vi "Main.vi"() -> ()   [LabVIEW 2013]
uses:
  <vilib>/vision/Image Controls.llb/IMAQ Image.ctl
  Controls/Tip.ctl
  Controls/Track.ctl
  <vilib>/vision/NI_Vision_Development_Module.lvlib
panel:
  in  "Tip Matching Options":T1
  in  "Track Classifier":path
  in  "Tracks":T2[](array[typedef]) {"ROI Descriptor"."Contours"."Type" items=["No Selection", "Point", "Line", "Rectangle", "Oval", "Polygon", "Freehand Region", "Annulus", "Unused2", "Unused3", "Broken Line", "Freehand Line", "Rotated Rectangle"]; "Tip 2"."ROI Descriptor"."Contours"."Type" items=["No Selection", "Point", "Line", "Rectangle", "Oval", "Polygon", "Freehand Region", "Annulus", "Unused2", "Unused3", "Broken Line", "Freehand Line", "Rotated Rectangle"]; "Tip 2"."Point"."Y" format="%.2f"; "Tip 2"."Point"."X" format="%.2f"; "Tip 1"."ROI Descriptor"."Contours"."Type" items=["No Selection", "Point", "Line", "Rectangle", "Oval", "Polygon", "Freehand Region", "Annulus", "Unused2", "Unused3", "Broken Line", "Freehand Line", "Rotated Rectangle"]; "Tip 1"."Point"."Y" format="%.2f"; "Tip 1"."Point"."X" format="%.2f"}
  in  "Flattened Stack":T6
  in  "Tip Classifier":path
  in  "Tips":T3[](array[typedef]) {"ROI Descriptor"."Contours"."Type" items=["No Selection", "Point", "Line", "Rectangle", "Oval", "Polygon", "Freehand Region", "Annulus", "Unused2", "Unused3", "Broken Line", "Freehand Line", "Rotated Rectangle"]; "Point"."Y" format="%.2f"; "Point"."X" format="%.2f"}
  in  "Tab Control":enum32{"Tip Extraction", "Track Extraction"}(tab)
  in  "Classify Tips":bool
  in  "Find Potential Tips":bool
  out "Progress":u8(slide) scale=0.0..100.0
  in  "Save Samples":bool
  in  "Reset":bool
  in  "Process AVI":bool
  in  "Process Directory":bool
  out "Currently Processing:":string
  in  "Stop":bool
  in  "Skip":bool
  out "Files to Process":i32
  in  "Tip Destination":path=path "C:/Users/Andrew/Documents/Apatite to Zircon Code/Track Finding/Tip Images/Tips/unprocessed"
  in  "Non-tip Destination":path=path "C:/Users/Andrew/Documents/Apatite to Zircon Code/Track Finding/Tip Images/Non-Tips/unprocessed"
  out "Tip Image":T6(plugin-control)
  in  "Save Track Samples":bool
  in  "Skip Track":bool
  in  "Track -":bool
  in  "Track +":bool
  in  "Classify Tracks":bool
  in  "Match Tips":bool
  in  "Track Destination":path=path "C:/Users/Andrew/Documents/Apatite to Zircon Code/Track Finding/Track Images/Tracks/unprocessed"
  in  "Non-track Destination":path=path "C:/Users/Andrew/Documents/Apatite to Zircon Code/Track Finding/Track Images/Non-tracks/unprocessed"
  out "Selected Track":T6(plugin-control)
  in  "Candidate Tracks":i32(listbox)
  out "File Index":i32
  in  "Image Array":T6[](array[typedef])
  in  "Filenames":path[](array[path])
  in  "Frame":i32(slide)
  in  "Current Image":T6(plugin-control)
  out "error out":errorcluster
  in  "error in (no error)":errorcluster
  # "AVI Processing"
  # "Extracted Samples"
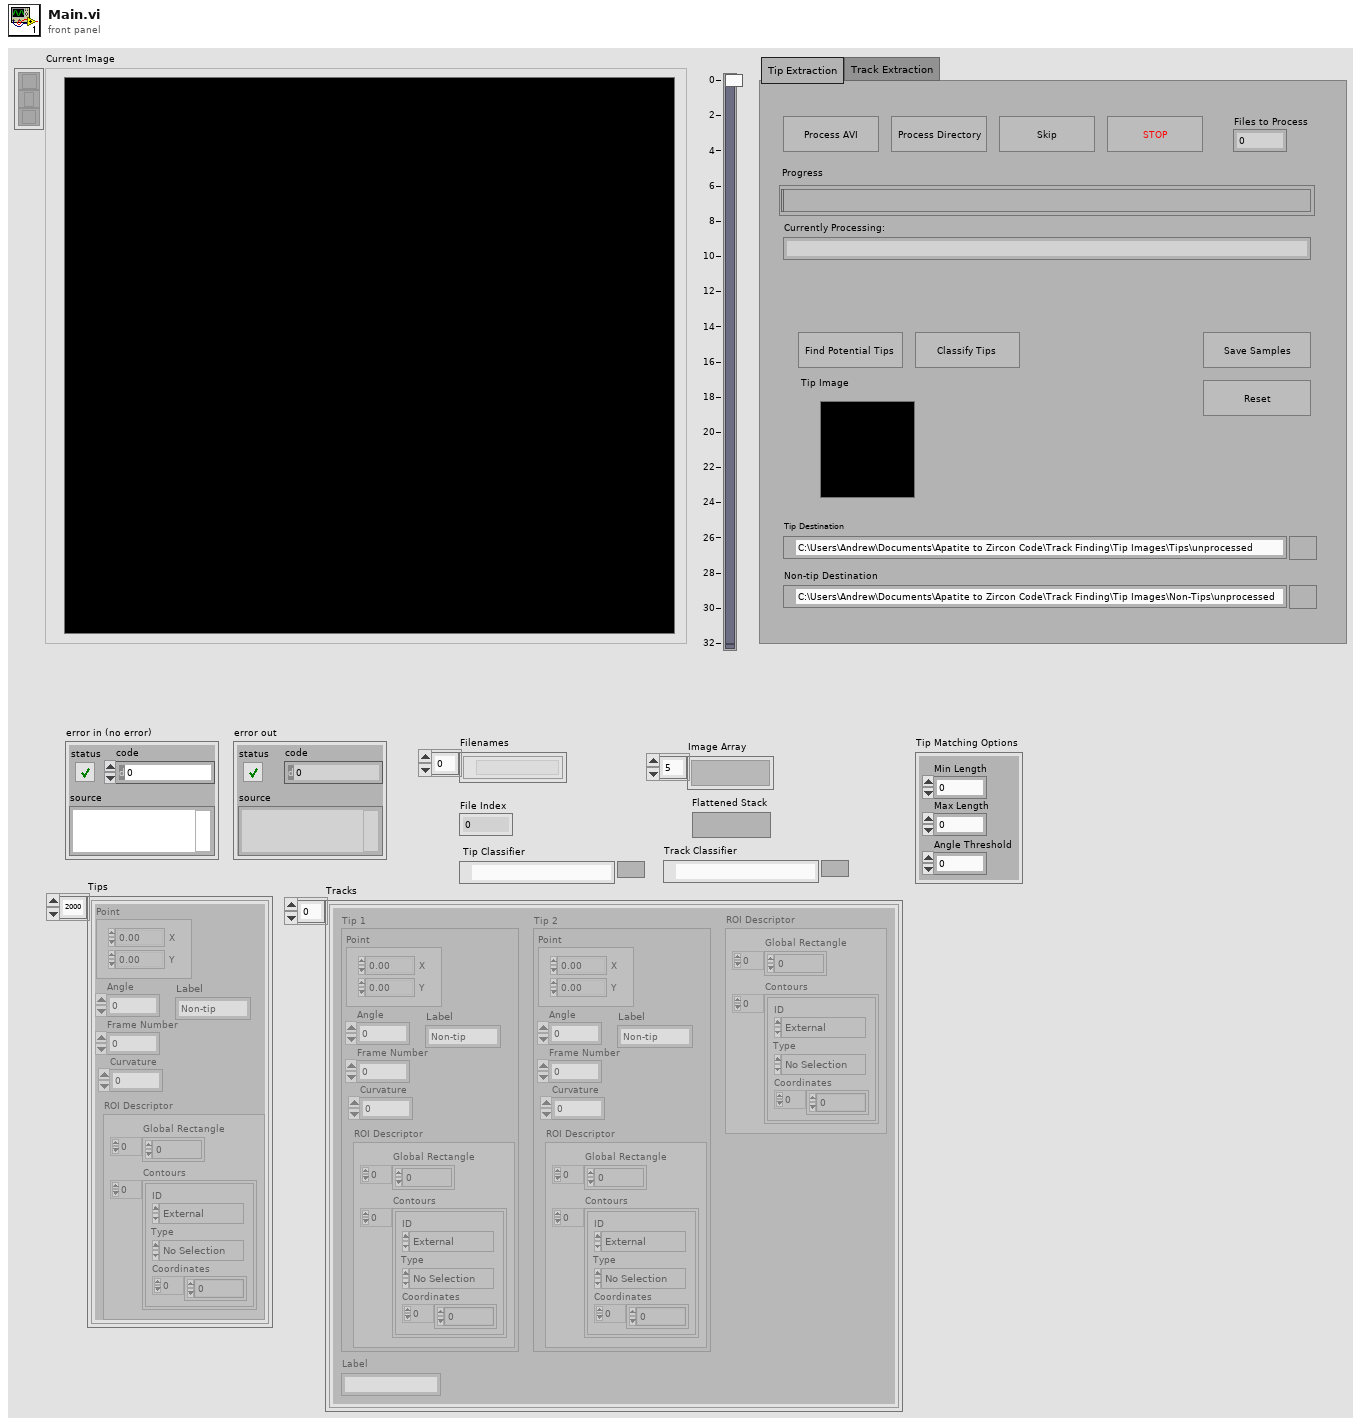
[diagram p1: front panel]
types:
  T1 = cluster{"Min Length":dbl, "Max Length":dbl, "Angle Threshold":dbl}
  T2 = typedef "Track.ctl" = cluster{"Tip 1":T3, "Tip 2":T3, "Label":string, "ROI Descriptor":T5}
  T3 = typedef "Tip.ctl" = cluster{"Point":T4, "Angle":dbl, "Frame Number":i32, "ROI Descriptor":T5, "Curvature":dbl, "Label":string}
  T4 = typedef "IMAQ Point" = cluster{"X":sgl, "Y":sgl}
  T5 = typedef "ROI Descriptor" = cluster{"Global Rectangle":i32[], "Contours":cluster{"ID":enum32{"External", "Internal"}, "Type":u32, "Coordinates":i32[]}[]}
  T6 = typedef "IMAQ Image.ctl" = refnum<image>
  T7 = enum8{"Enabled", "Disabled", "Disabled and Grayed Out"}
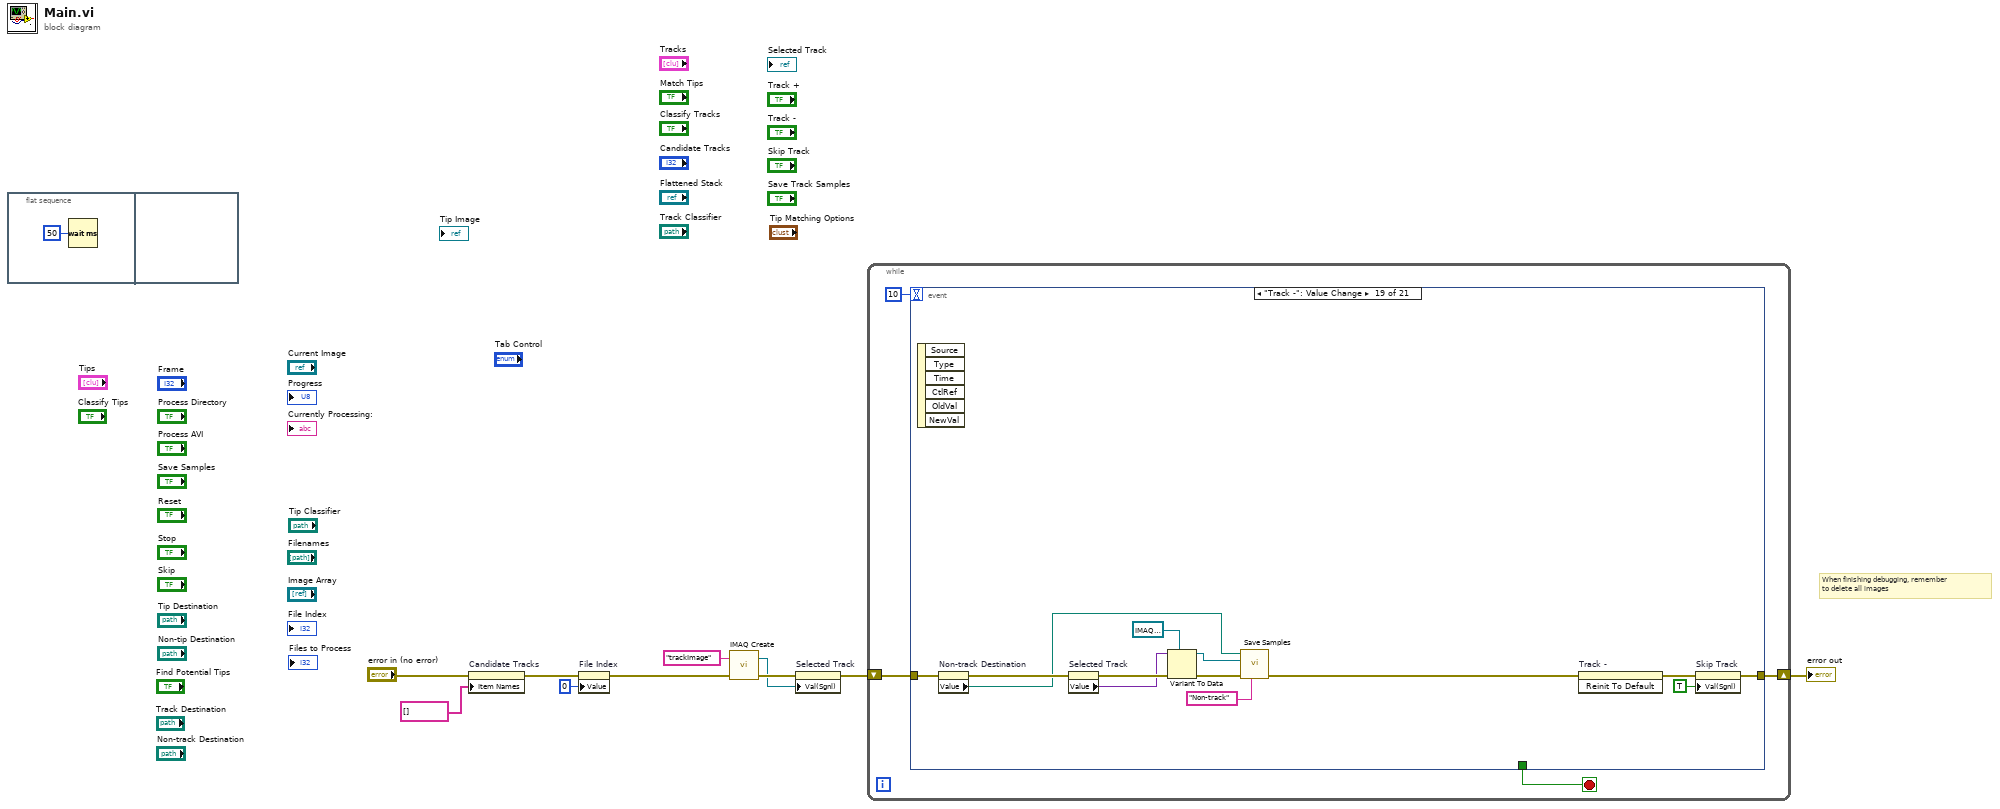
[diagram p0: block diagram]
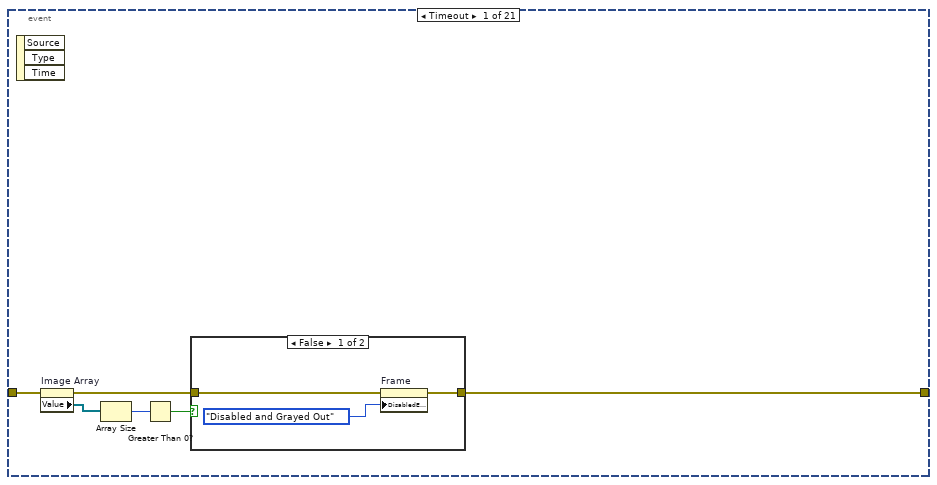
[diagram p2: hidden frame]
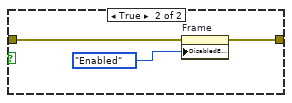
[diagram p3: hidden frame]
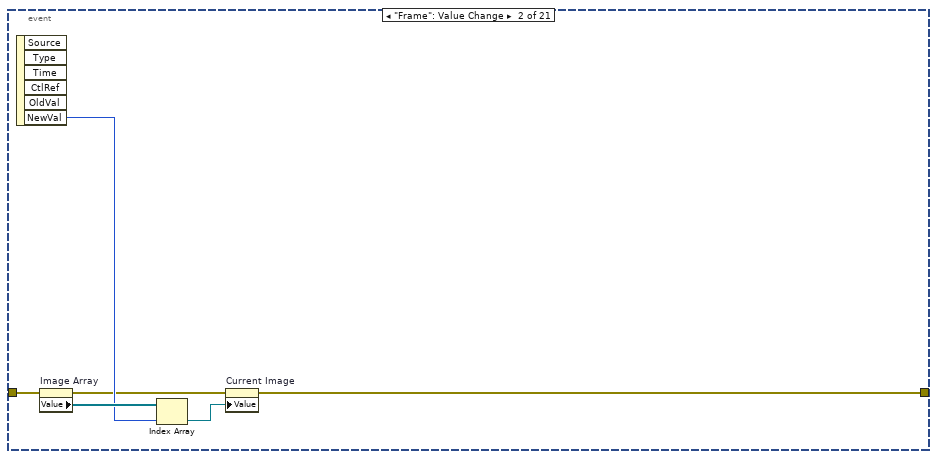
[diagram p4: hidden frame]
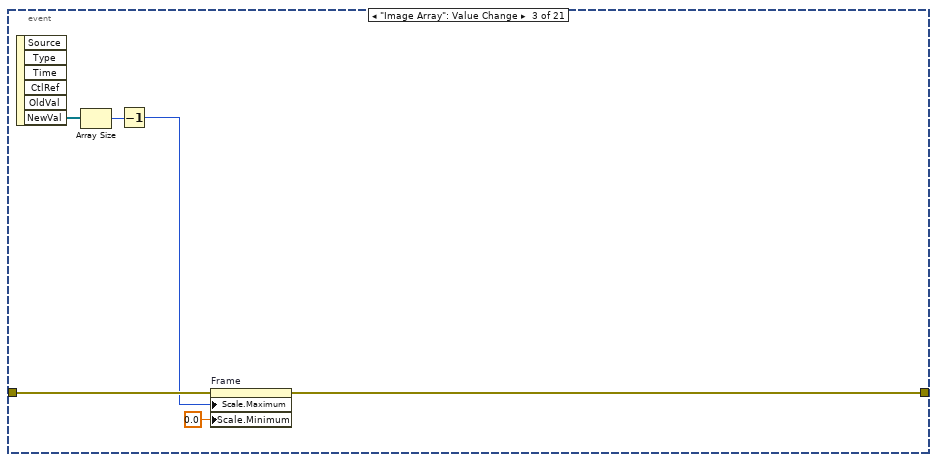
[diagram p5: hidden frame]
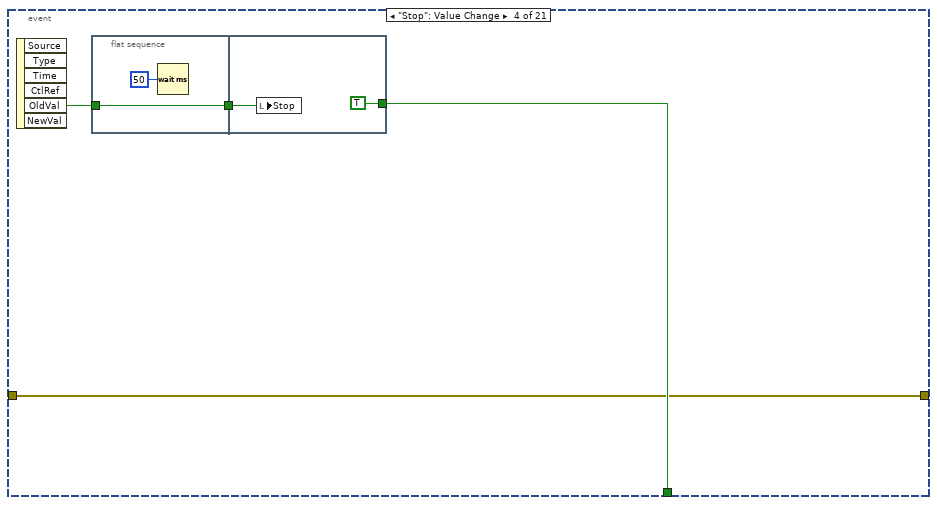
[diagram p6: hidden frame]
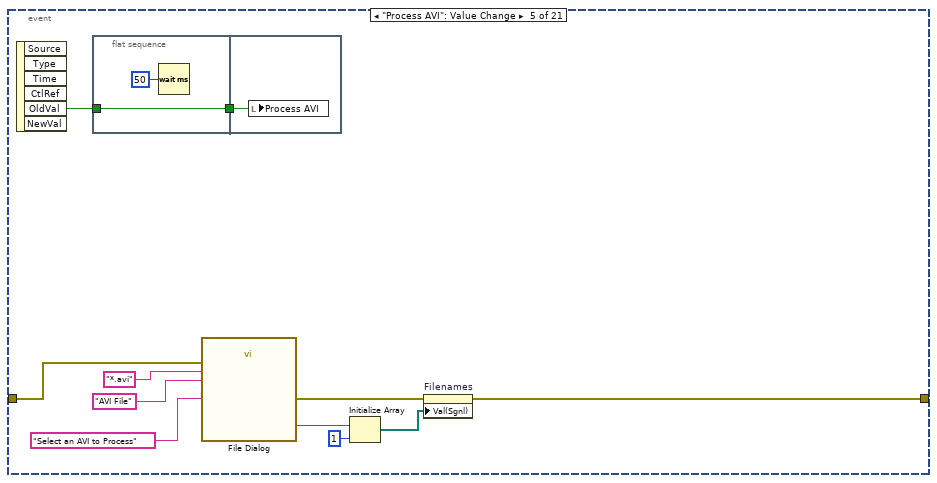
[diagram p7: hidden frame]
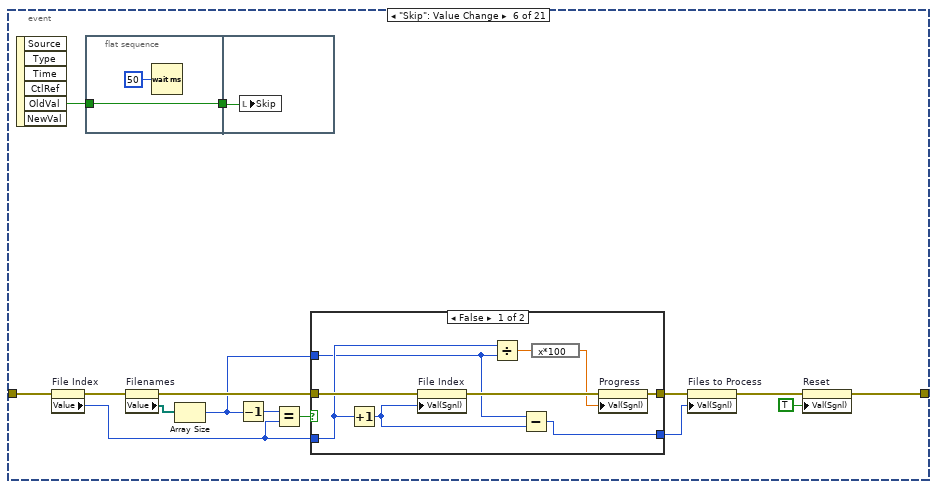
[diagram p8: hidden frame]
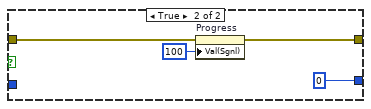
[diagram p9: hidden frame]
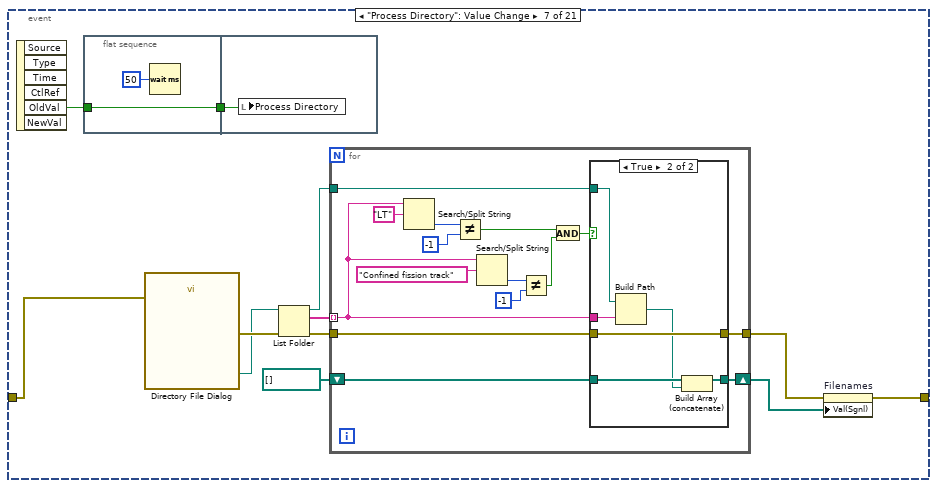
[diagram p10: hidden frame]
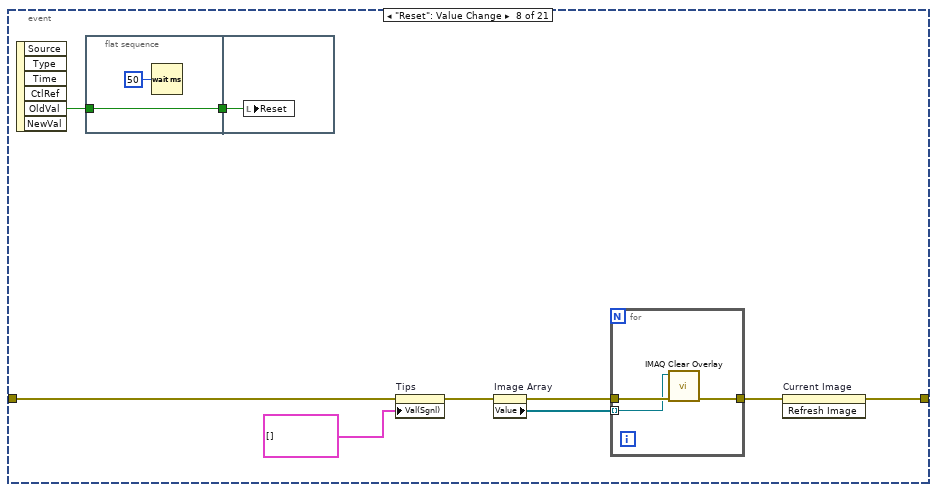
[diagram p12: hidden frame]
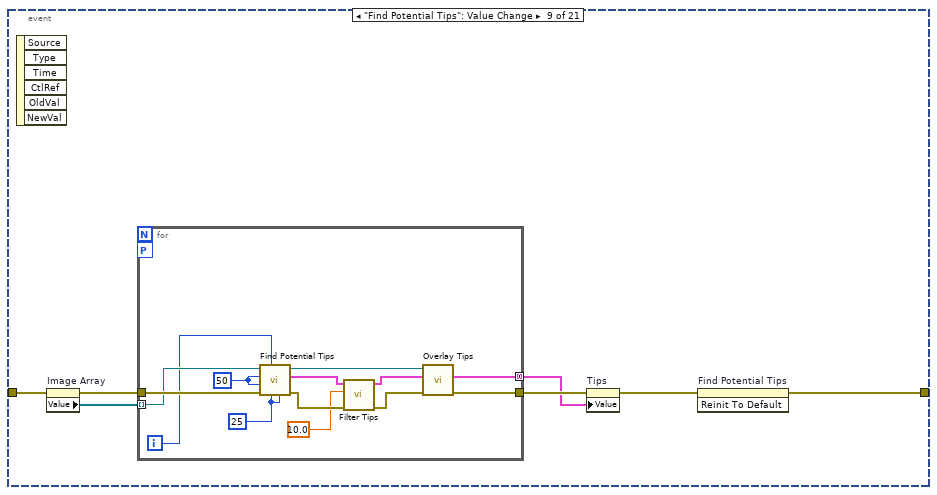
[diagram p13: hidden frame]
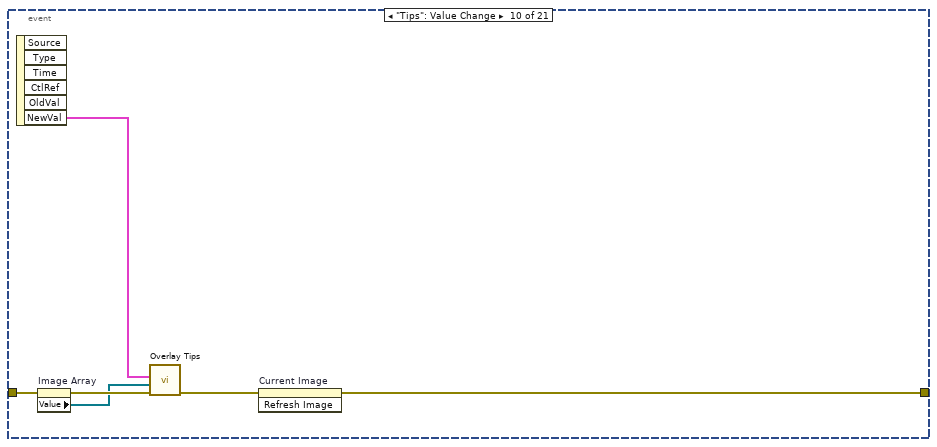
[diagram p14: hidden frame]
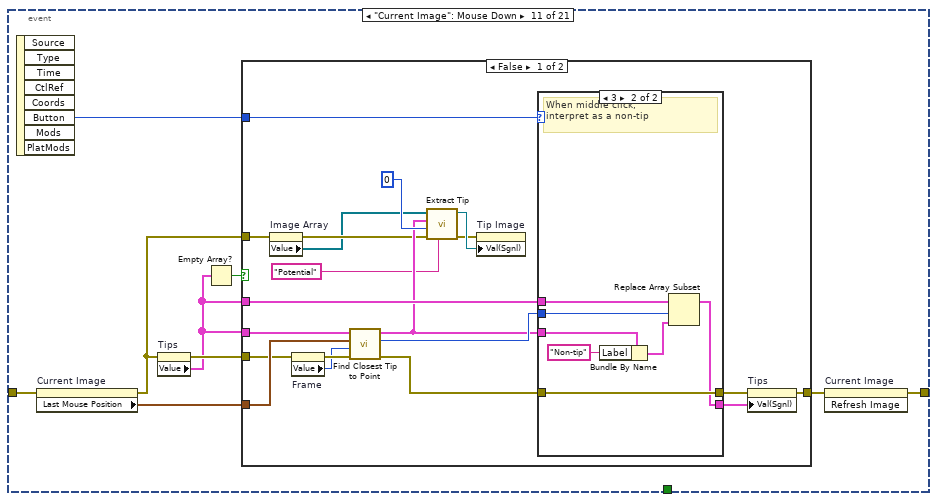
[diagram p15: hidden frame]
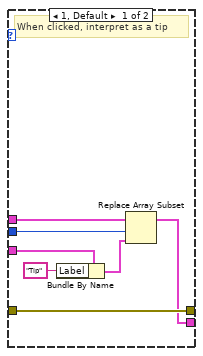
[diagram p16: hidden frame]
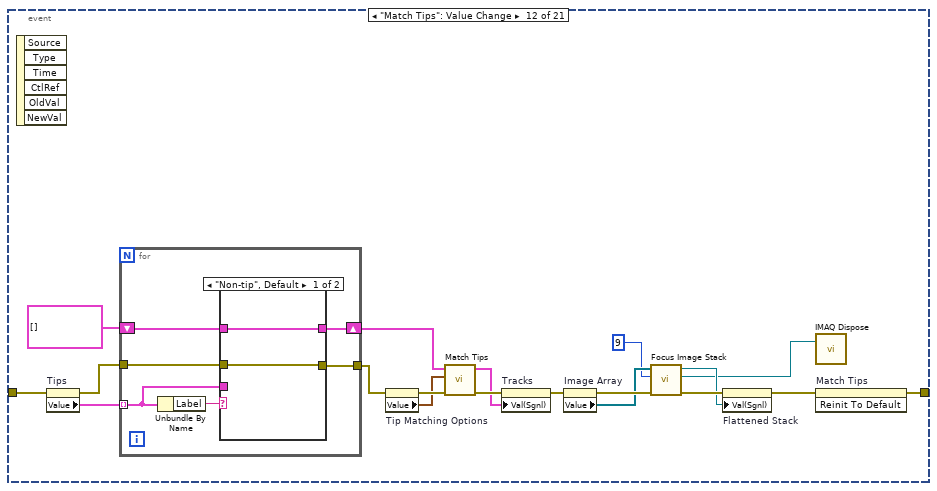
[diagram p18: hidden frame]
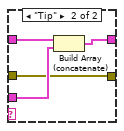
[diagram p19: hidden frame]
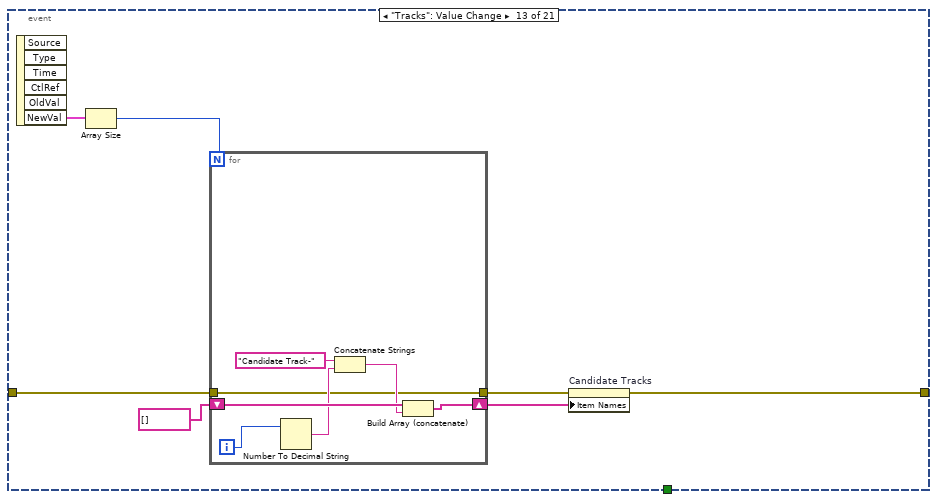
[diagram p20: hidden frame]
diagram:
  # "When finishing debugging, remember \nto delete all images"
  n1 = flat-sequence {
    frame #0 {
      n2 = Wait (ms)(milliseconds to wait=u32 50) -> ()  [unwired: 1 out]
    }
    frame #1 {
    }
  }
  n3 = property on="Candidate Tracks" class="LstBox (strict)"(error in="error in (no error)", "Item Names"=string[] []) -> (error out=w7:errorcluster)  [unwired: 1 in, 1 out]
  n4 = property on="File Index" class="DigNum (strict)"(error in=w7, "Value"=0 ("File Index")) -> (error out=w4:errorcluster)  [unwired: 1 in, 1 out]
  n5 = call "IMAQ Create"("Image Name"="trackImage", "error in (no error)"=w4) -> ("New Image"=w2:T6, "error out"=w3:errorcluster)  [unwired: 3 in]
  n6 = property on="Selected Track" class="ImageControl"(error in=w3, "Val(Sgnl)"=w2) -> (error out=w1:errorcluster)  [unwired: 1 in, 1 out]
  n7 = while {
    shift-right: [w13] -> w10
    shift-left: w1 -> [w14]
    stop <- w15 stop-if-true
    n8 = event shown="[18] \"Track -\": Value Change" {
      selector: _ -> [_ _ _ _ _ _ _ _ _ _ _ _ _ _ _ _ _ _ _ _ _]
      dyn-events: _ -> [_ _ _ _ _ _ _ _ _ _ _ _ _ _ _ _ _ _ _ _ _]
      timeout: 10 -> [_ _ _ _ _ _ _ _ _ _ _ _ _ _ _ _ _ _ _ _ _]
      tunnel: [_ _ _ w41 _ _ _ _ _ _ _ _ _ _ _ _ _ _ _ _ _] -> w15
      tunnel: w14 -> [w21 w33 w39 w40 w56 w74 w102 w132 w152 w171 w180 w231 w248 w279 w289 w304 w317 w364 w377 w386 w394]
      tunnel: [w16 w28 w35 w40 w49 w63 w97 w134 w146 w166 w177 w234 w249 w266 w280 w305 w319 w367 w380 w381 w387] -> w13
      event Timeout {
        n9 = event-data() -> ()  [unwired: 1 in, 3 out]
        n10 = property on="Image Array" class="Arr (strict)"(error in=w21) -> (error out=w17:errorcluster, "Value"=w20:T6[])  [unwired: 1 in, 1 out]
        n11 = Array Size(array=w20) -> (size(s)=w19:i32)
        n12 = Greater Than 0?(x=w19) -> (x > 0?=w18:bool)
        n13 = case shown="False" w18 {
          tunnel: w17 -> [w24 w26]
          tunnel: [w23 w25] -> w16
          frame False {
            n14 = property on="Frame" class="Slide (strict)"(error in=w24, "DisabledEnum"=T7."Disabled and Grayed Out" ("Disabled")) -> (error out=w23:errorcluster)  [unwired: 1 in, 1 out]
          }
          frame True {
            n15 = property on="Frame" class="Slide (strict)"(error in=w26, "DisabledEnum"=T7."Enabled" ("Disabled")) -> (error out=w25:errorcluster)  [unwired: 1 in, 1 out]
          }
        }
      }
      event "Frame": Value Change {
        n16 = event-data() -> ("NewVal"=w31:i32)  [unwired: 1 in, 5 out]
        n17 = property on="Image Array" class="Arr (strict)"(error in=w33) -> (error out=w30:errorcluster, "Value"=w32:T6[])  [unwired: 1 in, 1 out]
        n18 = Index Array(array=w32, index=w31) -> (element=w29:T6)
        n19 = property on="Current Image" class="ImageControl"(error in=w30, "Value"=w29) -> (error out=w28:errorcluster)  [unwired: 1 in, 1 out]
      }
      event "Image Array": Value Change {
        n20 = event-data() -> ("NewVal"=w38:T6[])  [unwired: 1 in, 5 out]
        n21 = Array Size(array=w38) -> (size(s)=w37:i32)
        n22 = Decrement(x=w37) -> (x-1=w36:i32)
        n23 = property on="Frame" class="Slide (strict)"(error in=w39, "Scale.Maximum"=w36, "Scale.Minimum"=0.0 ("Scale.Range:Minimum")) -> (error out=w35:errorcluster)  [unwired: 1 in, 1 out]
      }
      event "Stop": Value Change {
        n24 = event-data() -> ("OldVal"=w43:bool)  [unwired: 1 in, 5 out]
        n25 = flat-sequence {
          tunnel: w43 -> [w44]
          tunnel: [w44] -> w42
          tunnel: w42 -> [w47]
          tunnel: [TRUE] -> w41
          frame #0 {
            n26 = Wait (ms)(milliseconds to wait=u32 50) -> ()  [unwired: 1 out]
          }
          frame #1 {
            n27 = local write "Stop"(w47) -> ()
          }
        }
      }
      event "Process AVI": Value Change {
        n28 = event-data() -> ("OldVal"=w58:bool)  [unwired: 1 in, 5 out]
        n29 = flat-sequence {
          tunnel: w58 -> [w59]
          tunnel: [w59] -> w57
          tunnel: w57 -> [w61]
          frame #0 {
            n30 = Wait (ms)(milliseconds to wait=u32 50) -> ()  [unwired: 1 out]
          }
          frame #1 {
            n31 = local write "Process AVI"(w61) -> ()
          }
        }
        n32 = call "File Dialog"("prompt"="Select an AVI to Process", "error in"=w56, "pattern (all files)"="*.avi", "pattern label"="AVI File") -> ("selected path"=w53:path, "error out"=w50:errorcluster)  [unwired: 8 in, 2 out]
        n33 = Initialize Array(w53, 1 ("dimension size")) -> (w51:path[])
        n34 = property on="Filenames" class="Arr (strict)"(error in=w50, "Val(Sgnl)"=w51) -> (error out=w49:errorcluster)  [unwired: 1 in, 1 out]
      }
      event "Skip": Value Change {
        n35 = event-data() -> ("OldVal"=w75:bool)  [unwired: 1 in, 5 out]
        n36 = property on="File Index" class="DigNum (strict)"(error in=w74) -> (error out=w73:errorcluster, "Value"=w69:i32)  [unwired: 1 in, 1 out]
        n37 = flat-sequence {
          tunnel: [w90] -> w76
          tunnel: w75 -> [w90]
          tunnel: w76 -> [w92]
          frame #0 {
            n38 = Wait (ms)(milliseconds to wait=u32 50) -> ()  [unwired: 1 out]
          }
          frame #1 {
            n39 = local write "Skip"(w92) -> ()
          }
        }
        n40 = property on="Filenames" class="Arr (strict)"(error in=w73) -> (error out=w71:errorcluster, "Value"=w72:path[])  [unwired: 1 in, 1 out]
        n41 = Array Size(array=w72) -> (size(s)=w67:i32)
        n42 = Decrement(x=w67) -> (x-1=w68:i32)
        n43 = Equal?(x=w68, y=w69) -> (x = y?=w70:bool)
        n44 = case shown="False" w70 {
          tunnel: w71 -> [w85 w89]
          tunnel: w69 -> [w79 _]
          tunnel: [w83 w88] -> w66
          tunnel: w67 -> [w77 _]
          tunnel: [w78 0] -> w65
          frame False {
            n45 = Increment(x=w79) -> (x+1=w80:i32)
            n46 = property on="File Index" class="DigNum (strict)"(error in=w85, "Val(Sgnl)"=w80) -> (error out=w84:errorcluster)  [unwired: 1 in, 1 out]
            n47 = Divide(x=w79, y=w77) -> (x/y=w82:dbl)
            n48 = Subtract(x=w77, y=w80) -> (x-y=w78:i32)
            n49 = expression code="x*100"(w82) -> (w81:dbl)
            n50 = property on="Progress" class="Slide (strict)"(error in=w84, "Val(Sgnl)"=w81) -> (error out=w83:errorcluster)  [unwired: 1 in, 1 out]
          }
          frame True {
            n51 = property on="Progress" class="Slide (strict)"(error in=w89, "Val(Sgnl)"=u8 100 ("Value (Signaling)")) -> (error out=w88:errorcluster)  [unwired: 1 in, 1 out]
          }
        }
        n52 = property on="Files to Process" class="DigNum (strict)"(error in=w66, "Val(Sgnl)"=w65) -> (error out=w64:errorcluster)  [unwired: 1 in, 1 out]
        n53 = property on="Reset" class="Bool (strict)"(error in=w64, "Val(Sgnl)"=TRUE ("Value (Signaling)")) -> (error out=w63:errorcluster)  [unwired: 1 in, 1 out]
      }
      event "Process Directory": Value Change {
        n54 = event-data() -> ("OldVal"=w104:bool)  [unwired: 1 in, 5 out]
        n55 = flat-sequence {
          tunnel: w104 -> [w128]
          tunnel: [w128] -> w103
          tunnel: w103 -> [w130]
          frame #0 {
            n56 = Wait (ms)(milliseconds to wait=u32 50) -> ()  [unwired: 1 out]
          }
          frame #1 {
            n57 = local write "Process Directory"(w130) -> ()
          }
        }
        n58 = call "Directory File Dialog"("error in"=w102) -> ("selected path"=w98:path, "error out"=w99:errorcluster)  [unwired: 11 in, 2 out]
        n59 = List Folder(path=w98, error in=w99) -> (path out=w96:path, filenames=w101:string[], error out=w100:errorcluster)  [unwired: 2 in, 1 out]
        n60 = for {
          tunnel: w101 -> [w108] mode=indexing
          tunnel: w100 -> [w114]
          shift-right: [w115] -> w94
          shift-left: path[] [] -> [w116]
          tunnel: [w113] -> w93
          tunnel: w96 -> [w112]
          n61 = Search/Split String(string=w108, search string/char (-)="LT") -> (offset of match=w119:i32)  [unwired: 1 in, 2 out]
          n62 = Not Equal?(x=w119, y=-1) -> (x != y?=w106:bool)
          n63 = Search/Split String(string=w108, search string/char (-)="Confined fission track") -> (offset of match=w109:i32)  [unwired: 1 in, 2 out]
          n64 = Not Equal?(x=w109, y=-1) -> (x != y?=w107:bool)
          n65 = And(x=w106, y=w107) -> (x .and. y?=w105:bool)
          n66 = case shown="True" w105 {
            tunnel: w116 -> [w120 w127]
            tunnel: [w120 w126] -> w115
            tunnel: w108 -> [_ w124]
            tunnel: w114 -> [w121 w125]
            tunnel: [w121 w125] -> w113
            tunnel: w112 -> [_ w123]
            frame False {
            }
            frame True {
              n67 = Build Path(base path=w123, name or relative path=w124) -> (appended path=w122:path)
              n68 = Build Array (concatenate)(w127, w122) -> (w126:path[])
            }
          }
        }
        n69 = property on="Filenames" class="Arr (strict)"(error in=w93, "Val(Sgnl)"=w94) -> (error out=w97:errorcluster)  [unwired: 1 in, 1 out]
      }
      event "Reset": Value Change {
        n70 = event-data() -> ("OldVal"=w139:bool)  [unwired: 1 in, 5 out]
        n71 = flat-sequence {
          tunnel: w139 -> [w143]
          tunnel: [w143] -> w138
          tunnel: w138 -> [w145]
          frame #0 {
            n72 = Wait (ms)(milliseconds to wait=u32 50) -> ()  [unwired: 1 out]
          }
          frame #1 {
            n73 = local write "Reset"(w145) -> ()
          }
        }
        n74 = property on="Tips" class="Arr (strict)"(error in=w132, "Val(Sgnl)"=T3[] [] ("Value (Signaling)")) -> (error out=w133:errorcluster)  [unwired: 1 in, 1 out]
        n75 = property on="Image Array" class="Arr (strict)"(error in=w133) -> (error out=w136:errorcluster, "Value"=w137:T6[])  [unwired: 1 in, 1 out]
        n76 = for {
          tunnel: w137 -> [w141] mode=indexing
          tunnel: w136 -> [w142]
          tunnel: [w140] -> w135
          n77 = call "IMAQ Clear Overlay"("error in (no error)"=w142, "Image"=w141) -> ("error out"=w140:errorcluster)  [unwired: 8 in, 1 out]
        }
        n78 = invoke on="Current Image" class="ImageControl" method="Refresh Image"(error in=w135) -> (error out=w134:errorcluster)  [unwired: 2 in, 2 out]
      }
      event "Find Potential Tips": Value Change {
        n79 = event-data() -> ()  [unwired: 1 in, 6 out]
        n80 = property on="Image Array" class="Arr (strict)"(error in=w152) -> (error out=w151:errorcluster, "Value"=w150:T6[])  [unwired: 1 in, 1 out]
        n81 = for {
          workers-P: _ -> [_]
          tunnel: w151 -> [w165]
          tunnel: w150 -> [w164] mode=indexing
          tunnel: [w154] -> w148 mode=concatenating
          tunnel: [w153] -> w149
          i -> [w163]
          w161 = 50 ("ROI Width")
          w162 = 25 ("dx")
          n82 = call "Find Potential Tips.vi"("dy"=w162, "dx"=w162, "Frame Number"=w163, "error in (no error)"=w165, "ROI Height"=w161, "ROI Width"=w161, "Image"=w164) -> ("error out"=w160:errorcluster, "Potential Tips"=w159:T3[], "Image out"=w155:T6)  [unwired: 2 in]
          n83 = call "Filter Tips.vi"("error in (no error)"=w160, "Duplicate Distance"=10.0, "Tips"=w159) -> ("error out"=w156:errorcluster, "Filtered Tips"=w157:T3[])  [unwired: 7 in]
          n84 = call "Overlay Tips.vi"("error in (no error)"=w156, "Tips"=w157, "Image"=w155) -> ("error out"=w153:errorcluster, "Tips out"=w154:T3[])  [unwired: 6 in, 1 out]
        }
        n85 = property on="Tips" class="Arr (strict)"(error in=w149, "Value"=w148) -> (error out=w147:errorcluster)  [unwired: 1 in, 1 out]
        n86 = invoke on="Find Potential Tips" class="Bool (strict)" method="Reinit To Default"(error in=w147) -> (error out=w146:errorcluster)  [unwired: 2 in, 2 out]
      }
      event "Tips": Value Change {
        n87 = event-data() -> ("NewVal"=w168:T3[])  [unwired: 1 in, 5 out]
        n88 = property on="Image Array" class="Arr (strict)"(error in=w171) -> (error out=w170:errorcluster, "Value"=w169:T6[])  [unwired: 1 in, 1 out]
        n89 = call "Overlay Tips.vi"("error in (no error)"=w170, "Image Array"=w169, "Tips"=w168) -> ("error out"=w167:errorcluster)  [unwired: 6 in, 2 out]
        n90 = invoke on="Current Image" class="ImageControl" method="Refresh Image"(error in=w167) -> (error out=w166:errorcluster)  [unwired: 2 in, 2 out]
      }
      event "Current Image": Mouse Down {
        n91 = event-data() -> ("Button"=w178:u16)  [unwired: 1 in, 7 out]
        n92 = property on="Current Image" class="ImageControl"(error in=w180) -> (error out=w172:errorcluster, "Last Mouse Position"=w179:cluster{"X":i32, "Y":i32})  [unwired: 1 in, 1 out]
        n93 = property on="Tips" class="Arr (strict)"(error in=w172) -> (error out=w175:errorcluster, "Value"=w173:T3[])  [unwired: 1 in, 1 out]
        n94 = Empty Array?(array=w173) -> (empty?=w174:bool)
        n95 = case shown="False" w174 {
          tunnel: w179 -> [w195 _]
          tunnel: w178 -> [w200 _]
          tunnel: [w199 w215] -> w176
          tunnel: w175 -> [w194 w215]
          tunnel: w173 -> [w196 _]
          tunnel: w173 -> [w190 _]
          tunnel: w172 -> [w184 _]
          frame False {
            n96 = property on="Image Array" class="Arr (strict)"(error in=w184) -> (error out=w182:errorcluster, "Value"=w181:T6[])  [unwired: 1 in, 1 out]
            n97 = property on="Frame" class="Slide (strict)"(error in=w194) -> (error out=w193:errorcluster, "Value"=w192:i32)  [unwired: 1 in, 1 out]
            n98 = call "Find Closest Tip to Point.vi"("error in (no error)"=w193, "Frame Number"=w192, "Point"=w195, "Tips"=w196) -> ("error out"=w191:errorcluster, "Tip Index"=w189:i32, "Tip"=w185:T3)  [unwired: 5 in]
            n99 = call "Extract Tip.vi"("Label"="Potential", "error in (no error)"=w182, "Tip Number"=0, "Tip"=w185, "Image Array"=w181) -> ("error out"=w186:errorcluster, "Tip Image"=w187:T6)  [unwired: 5 in]
            n100 = property on="Tip Image" class="ImageControl"(error in=w186, "Val(Sgnl)"=w187) -> ()  [unwired: 1 in, 2 out]
            n101 = case shown="3" w200 {
              tunnel: w191 -> [w207 w214]
              tunnel: [w207 w214] -> w198
              tunnel: [w201 w208] -> w197
              tunnel: w185 -> [w206 w209]
              tunnel: w190 -> [w204 w211]
              tunnel: w189 -> [w203 w210]
              frame 1, Default {
                # "When clicked, interpret as a tip"
                n102 = Bundle By Name(cluster=w206, "Label"="Tip") -> (w202:T3)
                n103 = Replace Array Subset(array=w204, new element=w202, index=w203) -> (w201:T3[])
              }
              frame 3 {
                # "When middle click, \ninterpret as a non-tip"
                n104 = Bundle By Name(cluster=w209, "Label"="Non-tip") -> (w213:T3)
                n105 = Replace Array Subset(array=w211, new element=w213, index=w210) -> (w208:T3[])
              }
            }
            n106 = property on="Tips" class="Arr (strict)"(error in=w198, "Val(Sgnl)"=w197) -> (error out=w199:errorcluster)  [unwired: 1 in, 1 out]
          }
          frame True {
          }
        }
        n107 = invoke on="Current Image" class="ImageControl" method="Refresh Image"(error in=w176) -> (error out=w177:errorcluster)  [unwired: 2 in, 2 out]
      }
      event "Match Tips": Value Change {
        n108 = event-data() -> ()  [unwired: 1 in, 6 out]
        n109 = property on="Tips" class="Arr (strict)"(error in=w231) -> (error out=w228:errorcluster, "Value"=w227:T3[])  [unwired: 1 in, 1 out]
        n110 = for {
          tunnel: w228 -> [w236]
          tunnel: w227 -> [w237] mode=indexing
          shift-right: [w238] -> w224
          shift-left: T3[] [] -> [w239]
          tunnel: [w235] -> w226
          n111 = Unbundle By Name(w237) -> ("Label"=w240:string)
          n112 = case shown="\"Non-tip\", Default" w240 {
            tunnel: w239 -> [w242 w246]
            tunnel: [w242 w245] -> w238
            tunnel: w237 -> [_ w244]
            tunnel: [w241 w243] -> w235
            tunnel: w236 -> [w241 w243]
            frame "Non-tip", Default {
            }
            frame "Tip" {
              n113 = Build Array (concatenate)(w246, w244) -> (w245:T3[])
            }
          }
        }
        n114 = property on="Tip Matching Options" class="Clust (strict)"(error in=w226) -> (error out=w230:errorcluster, "Value"=w229:T1)  [unwired: 1 in, 1 out]
        n115 = call "Match Tips.vi"("error in (no error)"=w230, "Tip Matching Options"=w229, "Tips"=w224) -> ("error out"=w233:errorcluster, "Tracks"=w232:T2[])  [unwired: 7 in]
        n116 = property on="Tracks" class="Arr (strict)"(error in=w233, "Val(Sgnl)"=w232) -> (error out=w223:errorcluster)  [unwired: 1 in, 1 out]
        n117 = property on="Image Array" class="Arr (strict)"(error in=w223) -> (error out=w222:errorcluster, "Value"=w221:T6[])  [unwired: 1 in, 1 out]
        n118 = call "Focus Image Stack.vi"("error in (no error)"=w222, "Kernel Size"=9, "Image Stack"=w221) -> ("error out"=w219:errorcluster, "Height Map"=w216:T6, "Focused Image"=w218:T6)  [unwired: 6 in]
        n119 = property on="Flattened Stack" class="IMAQImage (strict)"(error in=w219, "Val(Sgnl)"=w218) -> (error out=w217:errorcluster)  [unwired: 1 in, 1 out]
        n120 = call "IMAQ Dispose"("Image"=w216) -> ()  [unwired: 5 in, 1 out]
        n121 = invoke on="Match Tips" class="Bool (strict)" method="Reinit To Default"(error in=w217) -> (error out=w234:errorcluster)  [unwired: 2 in, 2 out]
      }
      event "Tracks": Value Change {
        n122 = event-data() -> ("NewVal"=w253:T2[])  [unwired: 1 in, 5 out]
        n123 = Array Size(array=w253) -> (size(s)=w252:i32)
        n124 = for {
          N: w252 -> [_]
          tunnel: w248 -> [w254]
          shift-right: [w255] -> w250
          shift-left: string[] [] -> [w258]
          tunnel: [w254] -> w251
          i -> [w259]
          n125 = Number To Decimal String(number=w259) -> (decimal integer string=w257:string)  [unwired: 1 in]
          n126 = Concatenate Strings("Candidate Track-" ("string"), w257) -> (w256:string)
          n127 = Build Array (concatenate)(w258, w256) -> (w255:string[])
        }
        n128 = property on="Candidate Tracks" class="LstBox (strict)"(error in=w251, "Item Names"=w250) -> (error out=w249:errorcluster)  [unwired: 1 in, 1 out]
      }
      event "Candidate Tracks": Value Change {
        n129 = event-data() -> ("NewVal"=w277:i32)  [unwired: 1 in, 5 out]
        n130 = property on="Tracks" class="Arr (strict)"(error in=w279) -> (error out=w276:errorcluster, "Value"=w278:T2[])  [unwired: 1 in, 1 out]
        n131 = Index Array(array=w278, index=w277) -> (element=w271:T2)
        n132 = Unbundle By Name(w271) -> ("ROI Descriptor"=w269:T5)
        n133 = property on="Image Array" class="Arr (strict)" props=["Value"](error in=w276) -> (error out=w275:errorcluster)  [unwired: 1 in, 2 out]
        n134 = property on="Flattened Stack" class="IMAQImage (strict)"(error in=w275) -> (error out=w274:errorcluster, "Value"=w273:T6)  [unwired: 1 in, 1 out]
        n135 = call "Overlay Track.vi"("error in (no error)"=w274, "Flattened Image"=w273, "Track"=w271) -> ("error out"=w272:errorcluster, "Image out"=w270:T6)  [unwired: 7 in]
        n136 = property on="Current Image" class="ImageControl"(error in=w272, "Val(Sgnl)"=w270) -> (error out=w265:errorcluster)  [unwired: 1 in, 1 out]
        n137 = property on="Selected Track" class="ImageControl"(error in=w265) -> (error out=w263:errorcluster, "Value"=w264:variant)  [unwired: 1 in, 1 out]
        n138 = Variant To Data(type=T6 refnum ("Image Dst Out"), Variant=w264) -> (data=w261:T6)  [unwired: 1 in, 1 out]
        n139 = call-poly "IMAQ Extract Tetragon"("error in (no error)"=w263, "ROI Descriptor"=w269, "Image Dst"=w261, "Image Src"=w270) -> ("error out"=w268:errorcluster, "Image Dst Out"=w267:T6)  [unwired: 6 in]
        n140 = property on="Selected Track" class="ImageControl"(error in=w268, "Val(Sgnl)"=w267) -> (error out=w266:errorcluster)  [unwired: 1 in, 1 out]
      }
      event "Skip Track": Value Change {
        n141 = event-data() -> ()  [unwired: 1 in, 6 out]
        n142 = property on="Candidate Tracks" class="LstBox (strict)"(error in=w289) -> (error out=w288:errorcluster, "Value"=w283:i32)  [unwired: 1 in, 1 out]
        n143 = property on="Candidate Tracks" class="LstBox (strict)"(error in=w288) -> (error out=w286:errorcluster, "Item Names"=w287:string[])  [unwired: 1 in, 1 out]
        n144 = Array Size(array=w287) -> (size(s)=w285:i32)
        n145 = Decrement(x=w285) -> (x-1=w284:i32)
        n146 = Equal?(x=w284, y=w283) -> (x = y?=w282:bool)
        n147 = case shown="True" w282 {
          tunnel: w283 -> [w293 _]
          tunnel: w286 -> [w292 w294]
          tunnel: [w290 w294] -> w281
          frame False {
            n148 = Increment(x=w293) -> (x+1=w291:i32)
            n149 = property on="Candidate Tracks" class="LstBox (strict)"(error in=w292, "Val(Sgnl)"=w291) -> (error out=w290:errorcluster)  [unwired: 1 in, 1 out]
          }
          frame True {
          }
        }
        n150 = invoke on="Skip Track" class="Bool (strict)" method="Reinit To Default"(error in=w281) -> (error out=w280:errorcluster)  [unwired: 2 in, 2 out]
      }
      event "Classify Tips": Value Change {
        n151 = event-data() -> ()  [unwired: 1 in, 6 out]
        n152 = property on="Tips" class="Arr (strict)"(error in=w304) -> (error out=w299:errorcluster, "Value"=w300:T3[])  [unwired: 1 in, 1 out]
        n153 = property on="Tip Classifier" class="Path"(error in=w299) -> (error out=w298:errorcluster, "Value"=w295:path)  [unwired: 1 in, 1 out]
        n154 = property on="Image Array" class="Arr (strict)"(error in=w298) -> (error out=w297:errorcluster, "Value"=w296:T6[])  [unwired: 1 in, 1 out]
        n155 = call "Classify Tips.vi"("error in (no error)"=w297, "Image Array"=w296, "Classifier File"=w295, "Tips"=w300) -> ("error out"=w302:errorcluster, "Classified Tips"=w301:T3[])  [unwired: 6 in]
        n156 = property on="Tips" class="Arr (strict)"(error in=w302, "Val(Sgnl)"=w301) -> (error out=w303:errorcluster)  [unwired: 1 in, 1 out]
        n157 = invoke on="Classify Tips" class="Bool (strict)" method="Reinit To Default"(error in=w303) -> (error out=w305:errorcluster)  [unwired: 2 in, 2 out]
      }
      event "Save Samples": Value Change {
        n158 = event-data() -> ("OldVal"=w321:bool)  [unwired: 1 in, 5 out]
        n159 = property on="Tip Destination" class="Path"(error in=w317) -> (error out=w316:errorcluster, "Value"=w310:path)  [unwired: 1 in, 1 out]
        n160 = flat-sequence {
          tunnel: w321 -> [w352]
          tunnel: [w352] -> w320
          tunnel: w320 -> [w354]
          frame #0 {
            n161 = Wait (ms)(milliseconds to wait=u32 50) -> ()  [unwired: 1 out]
          }
          frame #1 {
            n162 = local write "Save Samples"(w354) -> ()
          }
        }
        n163 = property on="Non-tip Destination" class="Path"(error in=w316) -> (error out=w315:errorcluster, "Value"=w309:path)  [unwired: 1 in, 1 out]
        n164 = property on="Image Array" class="Arr (strict)"(error in=w315) -> (error out=w314:errorcluster, "Value"=w311:T6[])  [unwired: 1 in, 1 out]
        n165 = property on="Tips" class="Arr (strict)"(error in=w314) -> (error out=w313:errorcluster, "Value"=w312:T3[])  [unwired: 1 in, 1 out]
        n166 = for {
          tunnel: w313 -> [w332]
          tunnel: w312 -> [w327] mode=indexing
          tunnel: w311 -> [w331]
          tunnel: w310 -> [w325]
          tunnel: w309 -> [w324]
          tunnel: [w329] -> w307
          tunnel: [w322] -> w306
          n167 = Unbundle By Name(w327) -> ("Label"=w326:string)
          n168 = call "Extract Tip.vi"("Label"="Tip", "error in (no error)"=w332, "Tip Number"=0, "Tip"=w327, "Image Array"=w331) -> ("error out"=w323:errorcluster, "Tip Image"=w329:T6)  [unwired: 5 in]
          n169 = case shown="\"Non-tip\", Default" w326 {
            selector: w326 -> [w336 w349]
            tunnel: w329 -> [w340 w351]
            tunnel: w325 -> [_ w350]
            tunnel: w324 -> [w338 _]
            tunnel: w323 -> [w339 w348]
            tunnel: [w337 w347] -> w322
            frame "Non-tip", Default {
              n170 = Random Number (0-1)() -> (number: 0 to 1=w334:dbl)
              n171 = Less Or Equal?(x=w334, y=0.7) -> (x <= y?=w333:bool)
              n172 = case shown="True" w333 {
                tunnel: w340 -> [_ w346]
                tunnel: w339 -> [w341 w345]
                tunnel: w338 -> [_ w344]
                tunnel: [w341 w343] -> w337
                tunnel: w336 -> [_ w342]
                frame False {
                }
                frame True {
                  n173 = call "Save Samples.vi"("Type of Feature"=w342, "error in (no error)"=w345, "Image"=w346, "Destination Folder"=w344) -> ("error out"=w343:errorcluster)  [unwired: 7 in]
                }
              }
            }
            frame "Tip" {
              n174 = call "Save Samples.vi"("Type of Feature"=w349, "error in (no error)"=w348, "Image"=w351, "Destination Folder"=w350) -> ("error out"=w347:errorcluster)  [unwired: 7 in]
            }
          }
        }
        n175 = call "IMAQ Dispose"("Image"=w307, "error in (no error)"=w306) -> ("error out"=w308:errorcluster)  [unwired: 4 in]
        n176 = property on="Skip" class="Bool (strict)"(error in=w308, "Val(Sgnl)"=TRUE ("Value (Signaling)")) -> (error out=w319:errorcluster)  [unwired: 1 in, 1 out]
      }
      event "Track +": Value Change {
        n177 = event-data() -> ()  [unwired: 1 in, 6 out]
        n178 = property on="Track Destination" class="Path"(error in=w364) -> (error out=w360:errorcluster, "Value"=w357:path)  [unwired: 1 in, 1 out]
        n179 = property on="Selected Track" class="ImageControl"(error in=w360) -> (error out=w363:errorcluster, "Value"=w362:variant)  [unwired: 1 in, 1 out]
        n180 = Variant To Data(error in=w363, type=T6 refnum ("Selected Track"), Variant=w362) -> (data=w358:T6, error out=w359:errorcluster)
        n181 = call "Save Samples.vi"("Type of Feature"="Track", "error in (no error)"=w359, "Image"=w358, "Destination Folder"=w357) -> ("error out"=w355:errorcluster)  [unwired: 7 in]
        n182 = invoke on="Track +" class="Bool (strict)" method="Reinit To Default"(error in=w355) -> (error out=w365:errorcluster)  [unwired: 2 in, 2 out]
        n183 = property on="Skip Track" class="Bool (strict)"(error in=w365, "Val(Sgnl)"=TRUE ("Value (Signaling)")) -> (error out=w367:errorcluster)  [unwired: 1 in, 1 out]
      }
      event "Track -": Value Change {
        n184 = event-data() -> ()  [unwired: 1 in, 6 out]
        n185 = property on="Non-track Destination" class="Path"(error in=w377) -> (error out=w376:errorcluster, "Value"=w371:path)  [unwired: 1 in, 1 out]
        n186 = property on="Selected Track" class="ImageControl"(error in=w376) -> (error out=w374:errorcluster, "Value"=w373:variant)  [unwired: 1 in, 1 out]
        n187 = Variant To Data(error in=w374, type=T6 refnum ("Selected Track"), Variant=w373) -> (data=w370:T6, error out=w372:errorcluster)
        n188 = call "Save Samples.vi"("Type of Feature"="Non-track", "error in (no error)"=w372, "Image"=w370, "Destination Folder"=w371) -> ("error out"=w368:errorcluster)  [unwired: 7 in]
        n189 = invoke on="Track -" class="Bool (strict)" method="Reinit To Default"(error in=w368) -> (error out=w378:errorcluster)  [unwired: 2 in, 2 out]
        n190 = property on="Skip Track" class="Bool (strict)"(error in=w378, "Val(Sgnl)"=TRUE ("Value (Signaling)")) -> (error out=w380:errorcluster)  [unwired: 1 in, 1 out]
      }
      event "Filenames": Value Change {
        n191 = event-data() -> ("NewVal"=w384:path[])  [unwired: 1 in, 5 out]
        n192 = Array Size(array=w384) -> (size(s)=w382:i32)
        n193 = property on="File Index" class="DigNum (strict)"(error in=w386, "Val(Sgnl)"=0 ("Value (Signaling)")) -> (error out=w383:errorcluster)  [unwired: 1 in, 1 out]
        n194 = property on="Files to Process" class="DigNum (strict)"(error in=w383, "Val(Sgnl)"=w382) -> (error out=w381:errorcluster)  [unwired: 1 in, 1 out]
      }
      event "File Index": Value Change {
        n195 = event-data() -> ("NewVal"=w388:i32)  [unwired: 1 in, 5 out]
        n196 = property on="Filenames" class="Arr (strict)"(error in=w394) -> (error out=w390:errorcluster, "Value"=w389:path[])  [unwired: 1 in, 1 out]
        n197 = Index Array(array=w389, index=w388) -> (element=w393:path)
        n198 = call "Load New AVI.vi"("error in (no error)"=w390, "AVI Path"=w393) -> ("error out"=w392:errorcluster, "Image Array"=w391:T6[])  [unwired: 8 in]
        n199 = property on="Image Array" class="Arr (strict)"(error in=w392, "Val(Sgnl)"=w391) -> (error out=w387:errorcluster)  [unwired: 1 in, 1 out]
      }
    }
  }
  "error out" <- w10
